vi "Write PV_index.vi"(6 "Parameter":string="XQ01", 9 "Heater":string, 10 "EnumsAI":string[](array[string]), 11 "Heater in":refnum<class "Heater.lvclass">) -> (2 "Find":bool, 3 "Heater out":refnum<class "Heater.lvclass">)   [LabVIEW 2019, in "Heating.lvlib" / "Heater.lvclass"]
uses:
  Heater.lvclass
  Heater.lvclass/Heater.ctl
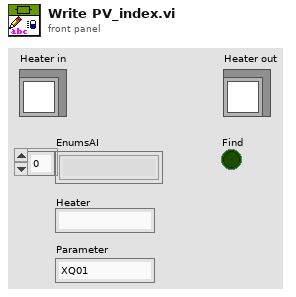
[diagram p1: front panel]
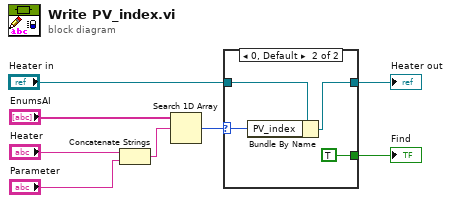
[diagram p0: block diagram]
diagram:
  n1 = Concatenate Strings("Heater", "Parameter") -> (w8:string)
  n2 = Search 1D Array(1D array="EnumsAI", element=w8) -> (index of element=w5:i32)  [unwired: 1 in]
  n3 = case shown="0, Default" w5 {
    selector: w5 -> [_ w11]
    tunnel: "Heater in" -> [w9 w13]
    tunnel: [w9 w12] -> w2
    tunnel: [_ TRUE] -> w4
    frame -1 {
    }
    frame 0, Default {
      n4 = Bundle By Name(cluster=w13, "PV_index"=w11) -> (w12:refnum<class "Heater.lvclass">)
    }
  }
  "Heater out" <- w2
  "Find" <- w4
